vi "Shutdown.vi"(11 "App Controller in":refnum<class "App Controller.lvclass">) -> (3 "App Controller out":refnum<class "App Controller.lvclass">)   [LabVIEW 2026, in "App Controller.lvclass"]
uses:
  App Controller.lvclass
  App Controller.lvclass/App Controller.ctl
  Core/Framework Engine/Framework Engine.lvclass
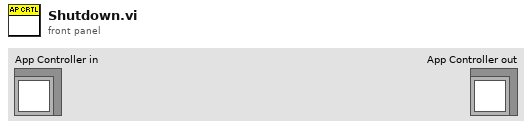
[diagram p1: front panel]
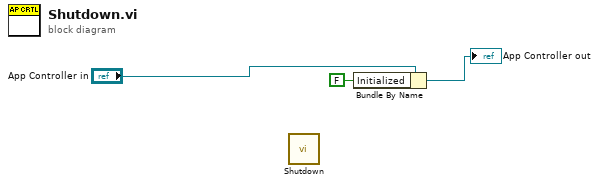
[diagram p0: block diagram]
diagram:
  n1 = call "Shutdown.vi"() -> ()  [unwired: 12 in]
  n2 = Bundle By Name(cluster="App Controller in", "Initialized"=FALSE) -> (→"App Controller out":refnum<class "App Controller.lvclass">)
